vi "Set Attribute.vi"(8 "error in (no error)":errorcluster, 9 "Value":variant, 10 "Name":string, 11 "AbstractData in":refnum<class "AbstractData.lvclass">) -> (0 "error out":errorcluster, 2 "replaced":bool, 3 "AbstractData out":refnum<class "AbstractData.lvclass">)   [LabVIEW 2014, in "AbstractData.lvclass"]
uses:
  AbstractData.lvclass
  AbstractData.lvclass/AbstractData.ctl
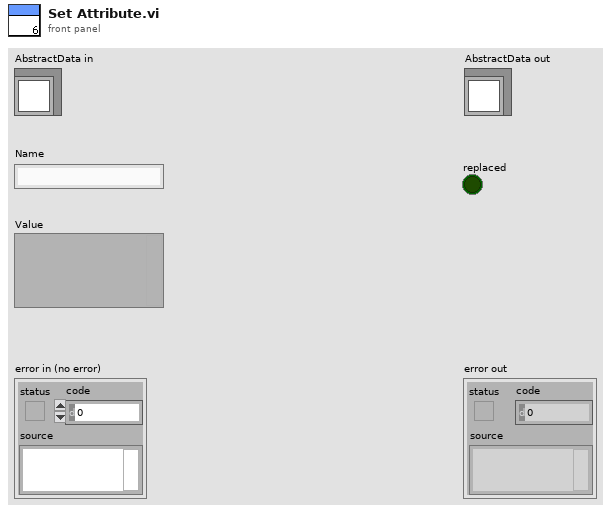
[diagram p1: front panel]
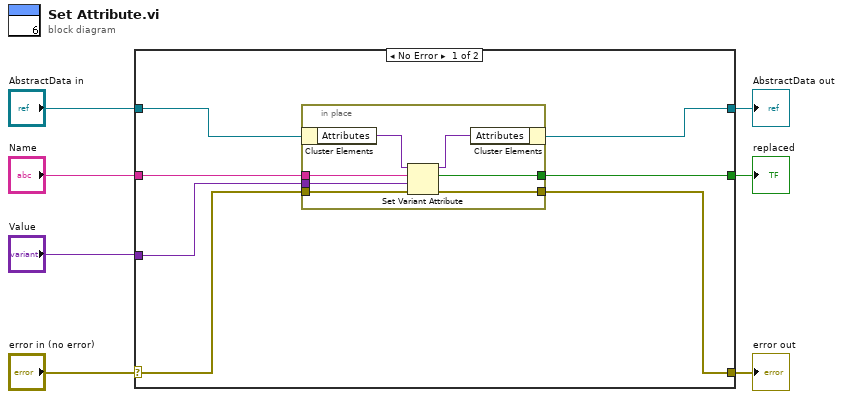
[diagram p0: block diagram]
diagram:
  n1 = case shown="No Error" "error in (no error)" {
    selector: "error in (no error)" -> [w11 w23]
    tunnel: [w9 w23] -> w6
    tunnel: [w13 w22] -> w4
    tunnel: "AbstractData in" -> [w14 w22]
    tunnel: "Value" -> [w10 _]
    tunnel: "Name" -> [w12 _]
    tunnel: [w8 _] -> w1
    frame No Error {
      n2 = in-place {
        in-place-border: w12 -> [w19]
        in-place-border: [w18] -> w9
        in-place-border: w11 -> [w17]
        in-place-border: w10 -> [w16]
        in-place-border: [w15] -> w8
        n3 = in-place-cluster #1(w14) -> ("Attributes"=w21:variant)
        n4 = Set Variant Attribute(Variant=w21, name=w19, value=w16, error in=w17) -> (Variant out=w20:variant, replaced=w15:bool, error out=w18:errorcluster)
        n5 = in-place-cluster #1("Attributes"=w20) -> (w13:refnum<class "AbstractData.lvclass">)
      }
    }
    frame Error {
    }
  }
  "error out" <- w6
  "AbstractData out" <- w4
  "replaced" <- w1
